vi "Query Cache Sizes.vi"(8 "error in (no error)":errorcluster, 11 "CPU Info in":refnum<class "CPU Hardware Info.lvclass">) -> (0 "error out":errorcluster, 2 "Caches":T1(array[cluster]), 3 "CPU Info out":refnum<class "CPU Hardware Info.lvclass">)   [LabVIEW 2017, in "Data Sharing Framework Engine.lvlib" / "CPU Hardware Info.lvclass"]
uses:
  CPU Hardware Info.lvclass
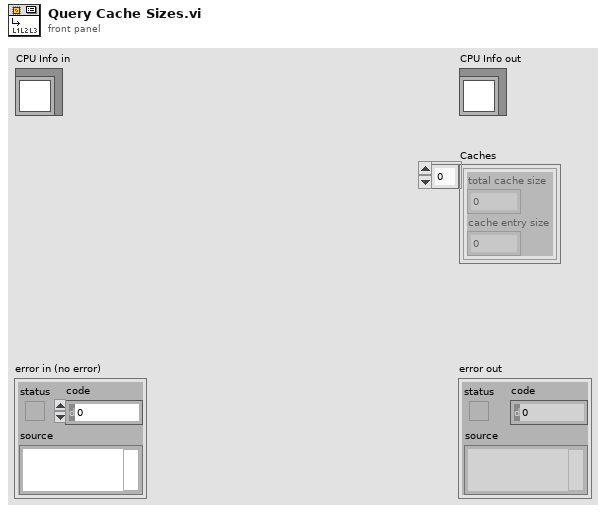
[diagram p1: front panel]
types:
  T1 = cluster{"total cache size":i32, "cache entry size":i32}[]
  T2 = cluster{"total cache size":i32, "cache entry size":i32}
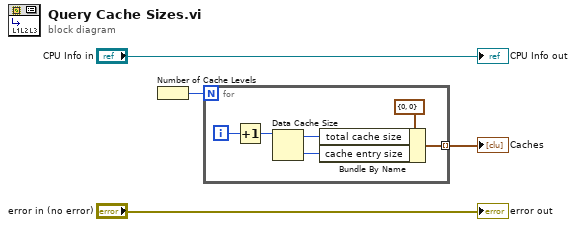
[diagram p0: block diagram]
diagram:
  n1 = Number of Cache Levels() -> (w2:i32)
  n2 = for {
    N: w2 -> [_]
    tunnel: [w7] -> w1 mode=indexing
    i -> [w6]
    n3 = Increment(x=w6) -> (x+1=w5:i32)
    n4 = Data Cache Size(0:w5) -> (4:w8:i32, 7:w9:i32)
    n5 = Bundle By Name(cluster=T2 {"total cache size"=0, "cache entry size"=0} ("caches"), "total cache size"=w8, "cache entry size"=w9) -> (w7:T2)
  }
  "Caches" <- w1
  "error out" <- "error in (no error)"
  "CPU Info out" <- "CPU Info in"
